vi "ProductUnit.vi"(5 "EndTime":timestamp, 6 "ScrappedTime":timestamp, 7 "StartTime":timestamp, 8 "error in (no error)":errorcluster, 9 "ManufacturingTime":timestamp, 10 "CreationTime":timestamp, 11 "ProductUnit in":refnum<class "ProductUnit.lvclass">) -> (0 "error out":errorcluster, 3 "Passed":bool)   [LabVIEW 2020]
uses:
  ProligentResultProcessor/ProductUnit/ProductUnit.lvclass
  ProligentResultProcessor/ProductUnit/SetProductUnitIdentifier.vi
  ProligentResultProcessor/ProductUnit/SetProductFullName.vi
  ProligentResultProcessor/ProductUnit/SetByManufacturer.vi
  ProligentResultProcessor/ProductUnit/SetCreationTime.vi
  ProligentResultProcessor/ProductUnit/SetManufacturingTime.vi
  ProligentResultProcessor/ProductUnit/SetScrappedTime.vi
  ProligentResultProcessor/ProductUnit/SetScrapped.vi
  ProligentResultProcessor/ProductUnit/GetProductUnitIdentifier.vi
  ProligentResultProcessor/ProductUnit/GetProductFullName.vi
  ProligentResultProcessor/ProductUnit/GetByManufacturer.vi
  ProligentResultProcessor/ProductUnit/GetCreationTime.vi
  ProligentResultProcessor/ProductUnit/GetManufacturingTime.vi
  ProligentResultProcessor/ProductUnit/GetScrappedTime.vi
  ProligentResultProcessor/ProductUnit/GetScrapped.vi
  ProligentResultProcessor/ProductUnit/GetCharacteristics.vi
  ProligentResultProcessor/ProductUnit/GetDocuments.vi
  ProligentResultProcessor/Model/Characteristic/Characteristic.lvclass
  ProligentResultProcessor/Model/Document/Document.lvclass
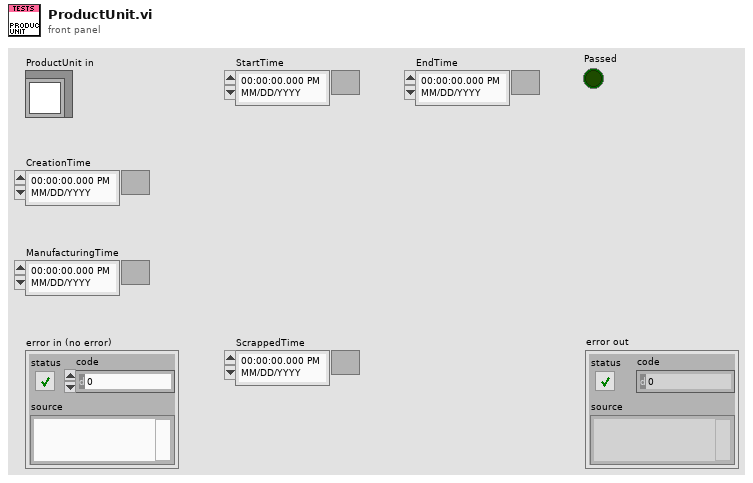
[diagram p1: front panel]
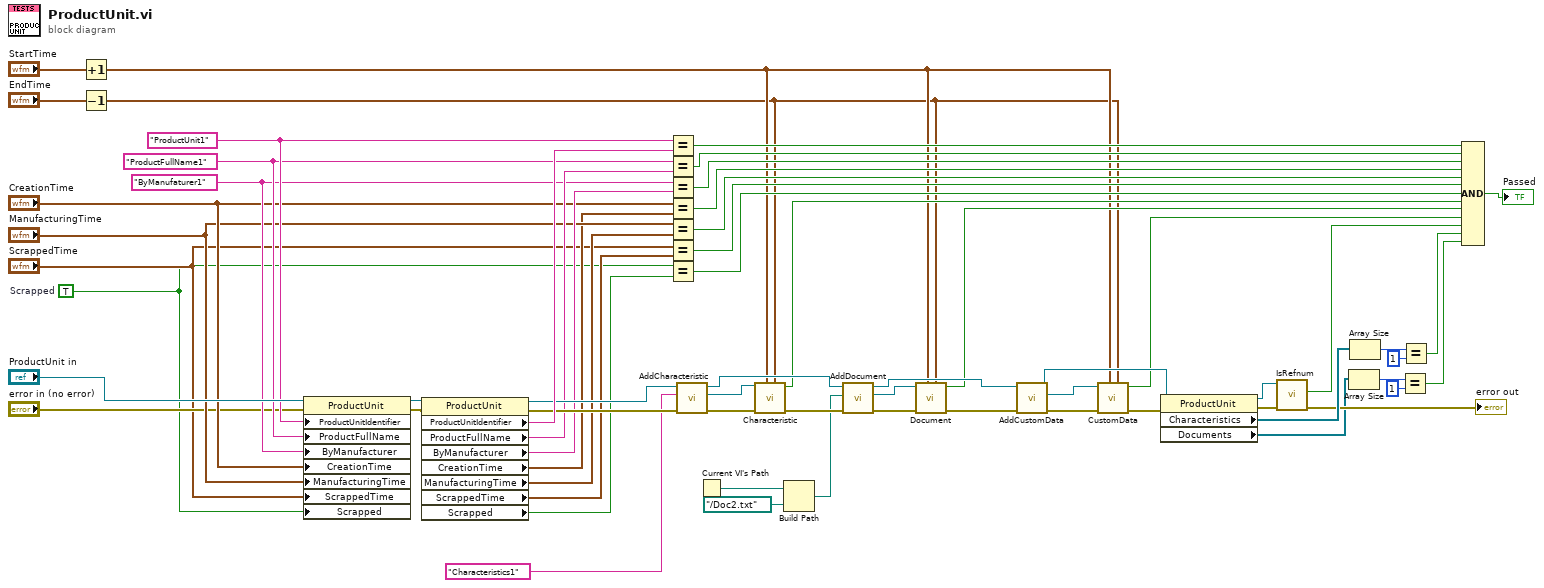
[diagram p0: block diagram]
diagram:
  w4 = TRUE  # Scrapped
  w41 = "ByManufaturer1"
  w42 = "ProductFullName1"
  w44 = "ProductUnit1"
  n1 = Increment(x="StartTime") -> (x+1=w11:timestamp)
  n2 = Decrement(x="EndTime") -> (x-1=w10:timestamp)
  n3 = property class="ProductUnit"(reference="ProductUnit in", error in="error in (no error)", "ProductUnitIdentifier"=w44, "ProductFullName"=w42, "ByManufacturer"=w41, "CreationTime"="CreationTime", "ManufacturingTime"="ManufacturingTime", "ScrappedTime"="ScrappedTime", "Scrapped"=w4) -> (reference out=w62:refnum<class "ProductUnit.lvclass">, error out=w61:errorcluster)
  n4 = property class="ProductUnit"(reference=w62, error in=w61) -> (reference out=w50:refnum<class "ProductUnit.lvclass">, error out=w51:errorcluster, "ProductUnitIdentifier"=w59:string, "ProductFullName"=w43:string, "ByManufacturer"=w40:string, "CreationTime"=w9:timestamp, "ManufacturingTime"=w8:timestamp, "ScrappedTime"=w7:timestamp, "Scrapped"=w5:bool)
  n5 = Equal?(x=w44, y=w59) -> (x = y?=w58:bool)
  n6 = Equal?(x=w42, y=w43) -> (x = y?=w57:bool)
  n7 = Equal?(x=w41, y=w40) -> (x = y?=w56:bool)
  n8 = Equal?(x="CreationTime", y=w9) -> (x = y?=w55:bool)
  n9 = Equal?(x="ManufacturingTime", y=w8) -> (x = y?=w54:bool)
  n10 = Equal?(x="ScrappedTime", y=w7) -> (x = y?=w53:bool)
  n11 = Equal?(x=w4, y=w5) -> (x = y?=w52:bool)
  n12 = call "AddCharacteristic.vi"("error in"=w51, "FullName"="Characteristics1", "ProcessRun in"=w50) -> ("error out"=w18:errorcluster, "Characteristics"=w16:refnum<class "Characteristic.lvclass">, "ProcessRun out"=w19:refnum<class "ProductUnit.lvclass">)  [unwired: 6 in]
  n13 = Current VI's Path() -> (path=w3:path)
  n14 = call "Characteristic.vi"("EndTime"=w10, "StartTime"=w11, "error in (no error)"=w18, "Characteristic in"=w16) -> ("error out"=w17:errorcluster, "Passed"=w15:bool)  [unwired: 6 in]
  n15 = Build Path(base path=w3, name or relative path=path "../Doc2.txt" ("FilePath")) -> (appended path=w1:path)
  n16 = call "AddDocument.vi"("error in"=w17, "FilePath"=w1, "ProductUnit in"=w19) -> ("error out"=w48:errorcluster, "Characteristics"=w13:refnum<class "Document.lvclass">, "ProductUnit out"=w47:refnum<class "ProductUnit.lvclass">)  [unwired: 6 in]
  n17 = call "Document.vi"("EndTime"=w10, "StartTime"=w11, "error in (no error)"=w48, "Characteristic in"=w13) -> ("error out"=w14:errorcluster, "Passed"=w12:bool)  [unwired: 6 in]
  n18 = call "AddCustomData.vi"("error in"=w14, "Defect in"=w47) -> ("error out"=w26:errorcluster, "CustomData"=w24:refnum<class "CustomData.lvclass">, "Defect out"=w45:refnum<class "ProductUnit.lvclass">)  [unwired: 7 in]
  n19 = call "CustomData.vi"("EndTime"=w10, "StartTime"=w11, "error in"=w26, "CustomData"=w24) -> ("error out"=w25:errorcluster, "Passed"=w21:bool)  [unwired: 6 in]
  n20 = property class="ProductUnit"(reference=w45, error in=w25) -> (reference out=w30:refnum<class "ProductUnit.lvclass">, error out=w37:errorcluster, "Characteristics"=w35:refnum<class "Characteristic.lvclass">[], "Documents"=w28:refnum<class "Document.lvclass">[])
  n21 = call "IsRefnum.vi"("error in"=w37, "ProductUnit in"=w30) -> ("error out"=→"error out":errorcluster, "IsRefnum"=w46:bool)  [unwired: 7 in, 1 out]
  n22 = Array Size(array=w28) -> (size(s)=w32:i32)
  n23 = Array Size(array=w35) -> (size(s)=w34:i32)
  n24 = Equal?(x=w32, y=1) -> (x = y?=w27:bool)
  n25 = Equal?(x=w34, y=1) -> (x = y?=w33:bool)
  n26 = Compound Arithmetic op=AND(w58, w57, w56, w55, w54, w53, w52, w15, w12, w21, w46, w33, w27) -> (→"Passed":bool)
